vi "CC Get Filter Names.vi"(8 "error in (no error)":errorcluster) -> (0 "error out":errorcluster, 2 "Wheel names":string[](array[string]), 3 "filter names":cluster{"Names":string[]}[](array[cluster]))   [LabVIEW 2024]
uses:
  Filter Wheel Object/Filter Wheel.lvclass
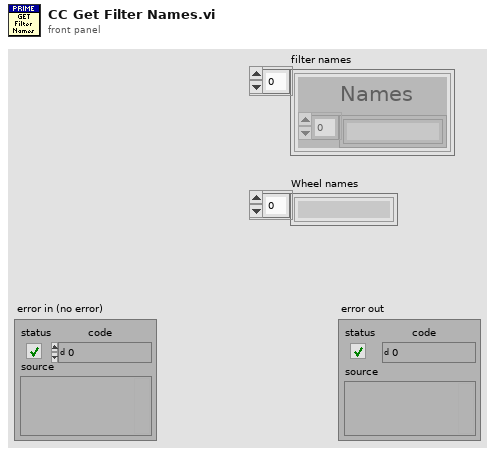
[diagram p1: front panel]
types:
  T1 = typedef "CC cluster Hardware Config.ctl" = cluster{"Installed Hardware":T2[]}
  T2 = typedef "CC cluster Device Index.ctl" = cluster{"Device Type Name":string, "Curr Device Name":string, "All Instances":string[]}
  T3 = typedef "Filter Wheel.lvclass/Filter Wheel configuration.ctl" = cluster{"Num Wheels":i32, "Filters":T4[], "Invalid Combinations":i32[][], "Addr":refnum<visa-resource-name>, "Name":string, "Simulate":bool, "Default Speed":u16, "Homing":T5[]}
  T4 = typedef "Filter Wheel.lvclass/Filter Wheel Details.ctl" = cluster{"Names":string[], "Relative Position":i32[], "Wheel Name":string, "Size":i32}
  T5 = typedef "Filter Wheel Arduino Homing cluster.ctl" = cluster{"Direction":bool, "Speed":i32, "Accel":i32, "Error Cnts":i32, "Homing Delta":i32}
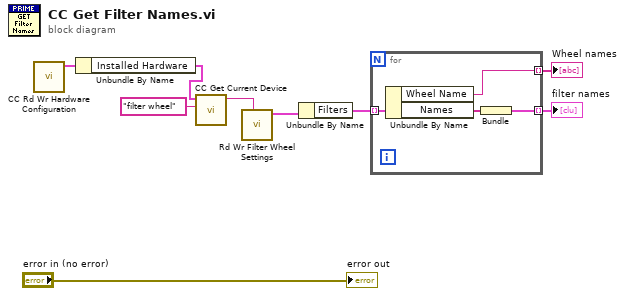
[diagram p0: block diagram]
diagram:
  n1 = call "CC Rd Wr Hardware Configuration.vi"() -> ("Hardware Config out"=w7:T1)  [unwired: 8 in, 3 out]
  n2 = Unbundle By Name(w7) -> ("Installed Hardware"=w6:T2[])
  n3 = call "CC Get Current Device.vi"("Device Type Name"="filter wheel", "Hardware.Installed Hardware"=w6) -> ("Curr Device Name"=w5:string)  [unwired: 7 in, 2 out]
  n4 = call "Rd Wr Filter Wheel Settings.vi"("Wheel Name"=w5) -> ("Filter Wheel Settings"=w4:T3)  [unwired: 9 in, 1 out]
  n5 = Unbundle By Name(w4) -> ("Filters"=w3:T4[])
  n6 = for {
    tunnel: w3 -> [w13] mode=indexing
    tunnel: [w11] -> w2 mode=indexing
    tunnel: [w10] -> w1 mode=indexing
    n7 = Unbundle By Name(w13) -> ("Wheel Name"=w10:string, "Names"=w12:string[])
    n8 = Bundle("Names"=w12) -> (w11:cluster{"Names":string[]})  [unwired: 1 in]
  }
  "filter names" <- w2
  "Wheel names" <- w1
  "error out" <- "error in (no error)"
